vi "Part 2.vi"(11 "Input":string) -> (3 "Output":i64)   [LabVIEW 2021]
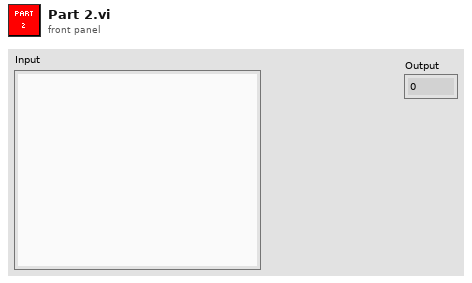
[diagram p1: front panel]
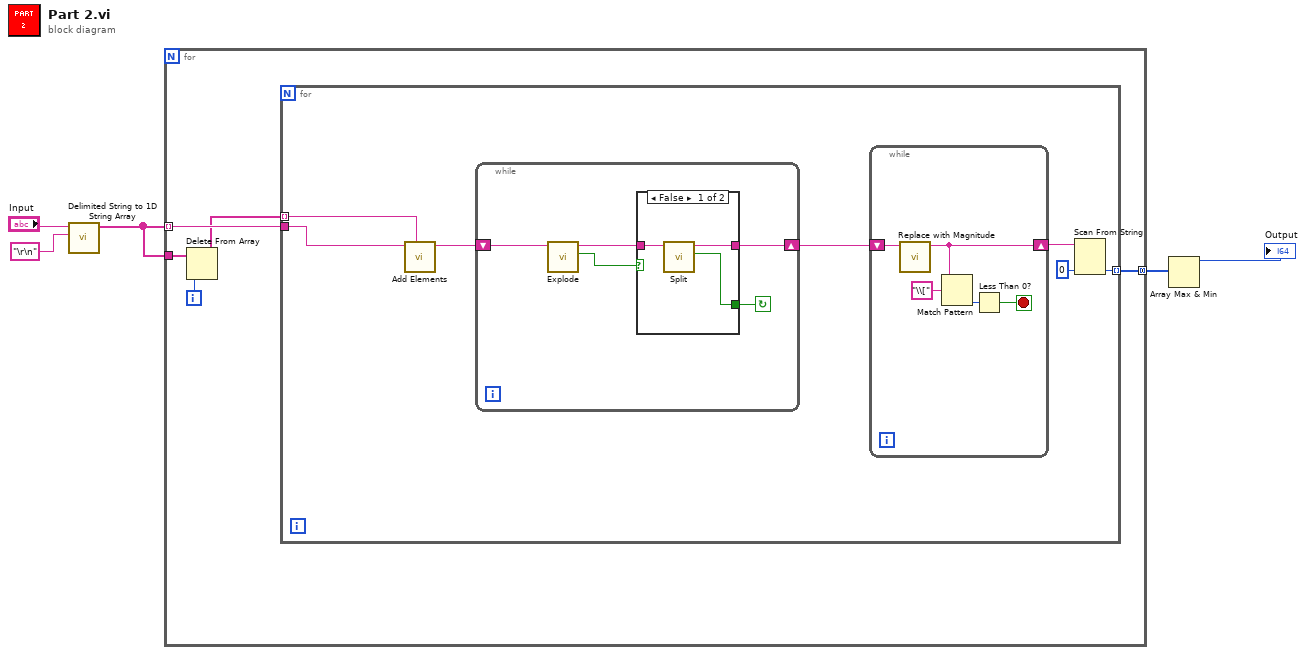
[diagram p0: block diagram]
diagram:
  n1 = call <vilib>:"Delimited String to 1D String Array.vi"("delimiter"="\r\n", "delimited string"="Input") -> ("string array"=w3:string[])  [unwired: 9 in]
  n2 = for {
    tunnel: w3 -> [w8] mode=indexing
    tunnel: w3 -> [w9]
    tunnel: [w6] -> w2 mode=concatenating
    i -> [w10]
    n3 = Delete From Array(array=w9, index=w10) -> (array with subset deleted=w7:string[])  [unwired: 1 in, 1 out]
    n4 = for {
      tunnel: w8 -> [w14]
      tunnel: w7 -> [w13] mode=indexing
      tunnel: [w12] -> w6 mode=indexing
      n5 = call "Add Elements.vi"("Element 2"=w13, "Element 1"=w14) -> ("Sum"=w11:string)  [unwired: 9 in]
      n6 = while {
        shift-right: [w22] -> w17
        shift-left: w11 -> [w20]
        stop <- w21 continue-if-true
        n7 = call "Explode.vi"("String In"=w20) -> ("Exploded?"=w18:bool, "String Out"=w19:string)  [unwired: 9 in]
        n8 = case shown="False" w18 {
          selector: w18 -> [_ w27]
          tunnel: [w25 w26] -> w22
          tunnel: [w24 w27] -> w21
          tunnel: w19 -> [w23 w26]
          frame False {
            n9 = call "Split.vi"("String In"=w23) -> ("Splitted?"=w24:bool, "String Out"=w25:string)  [unwired: 9 in]
          }
          frame True {
          }
        }
      }
      n10 = while {
        shift-right: [w28] -> w16
        shift-left: w17 -> [w29]
        stop <- w30 stop-if-true
        n11 = call "Replace with Magnitude.vi"("String In"=w29) -> ("String Out"=w28:string)  [unwired: 10 in]
        n12 = Match Pattern(string=w28, regular expression="\\[") -> (offset past match=w31:i32)  [unwired: 1 in, 3 out]
        n13 = Less Than 0?(x=w31) -> (x < 0?=w30:bool)
      }
      n14 = Scan From String(input string=w16, default 1=i64 0 ("Output")) -> (output 1=w12:i64)  [unwired: 3 in, 3 out]
    }
  }
  n15 = Array Max & Min(array=w2) -> (max value=→"Output":i64)  [unwired: 3 out]
